vi "onConnection.vi"(8 "error in (no error)":errorcluster, 11 "Connection in":refnum<class "Connection.lvclass">) -> (0 "error out":errorcluster, 3 "Connection out":refnum<class "Connection.lvclass">)   [LabVIEW 2013, in "Connection_GOSPL.lvlib" / "Connection.lvclass"]
uses:
  Connection.lvclass
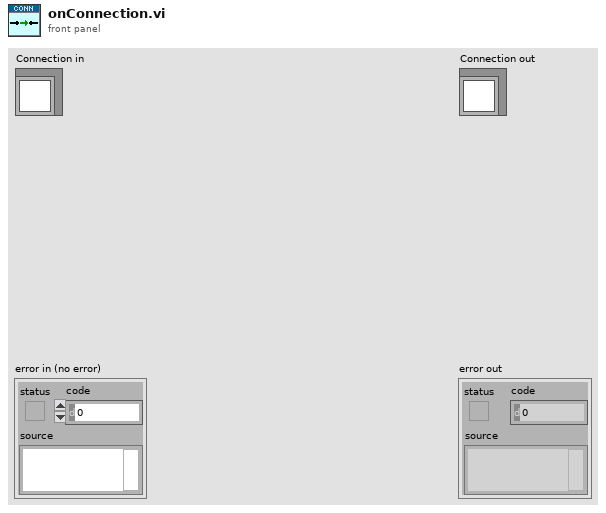
[diagram p1: front panel]
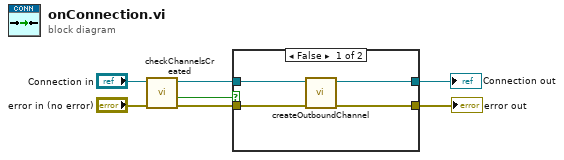
[diagram p0: block diagram]
diagram:
  n1 = call-dynamic "checkChannelsCreated.vi"("error in (no error)"="error in (no error)", "Connection in"="Connection in") -> ("error out"=w6:errorcluster, "outbound created"=w7:bool, "Connection out"=w1:refnum<class "Connection.lvclass">)  [unwired: 6 in, 1 out]
  n2 = case shown="False" w7 {
    tunnel: w6 -> [w10 w12]
    tunnel: [w9 w12] -> w2
    tunnel: w1 -> [w8 w13]
    tunnel: [w11 w13] -> w4
    frame False {
      n3 = call-dynamic "createOutboundChannel.vi"("error in (no error)"=w10, "Connection in"=w8) -> ("error out"=w9:errorcluster, "Connection out"=w11:refnum<class "Connection.lvclass">)  [unwired: 8 in]
    }
    frame True {
    }
  }
  "error out" <- w2
  "Connection out" <- w4
